vi "Destroy_Tree.vi"(8 "error in (no error)":errorcluster, 10 "Delete Tree Items? (F)":bool, 11 "Tree_LVOOP in":refnum<class "Tree Class.lvclass">) -> (0 "error out":errorcluster)   [LabVIEW 2012, in "Tree Tools.lvlib" / "Tree Class.lvclass"]
uses:
  Tree Class.lvclass
  Tree Class.lvclass/Tree Class.ctl
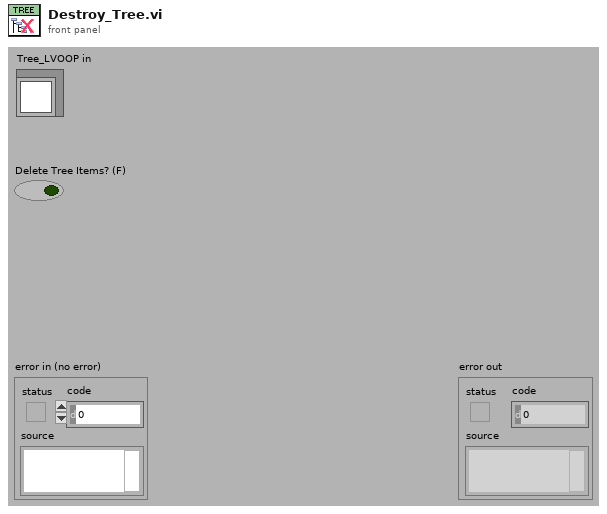
[diagram p1: front panel]
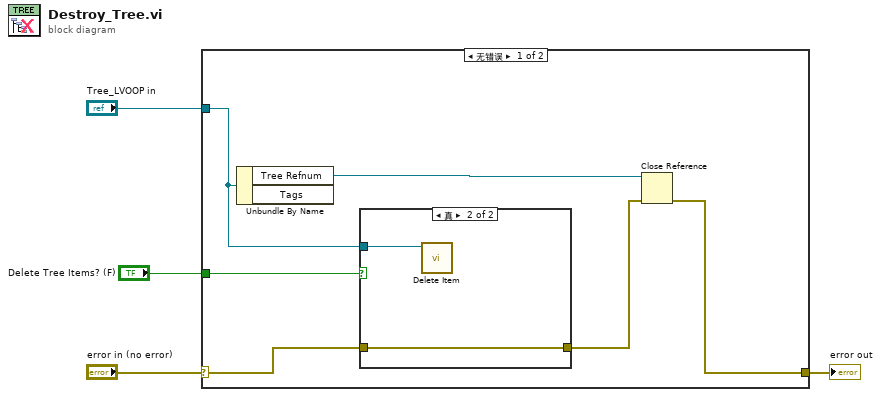
[diagram p0: block diagram]
diagram:
  n1 = case shown="无错误" "error in (no error)" {
    selector: "error in (no error)" -> [w7 w14]
    tunnel: [w9 w14] -> w3
    tunnel: "Tree_LVOOP in" -> [w5 _]
    tunnel: "Delete Tree Items? (F)" -> [w8 _]
    frame No Error {
      n2 = Unbundle By Name(w5) -> ("Tree Refnum"=w10:refnum<vi>)  [unwired: 1 out]
      n3 = case shown="真" w8 {
        tunnel: w7 -> [w11 w13]
        tunnel: [w11 w13] -> w6
        tunnel: w5 -> [_ w12]
        frame False {
        }
        frame True {
          n4 = call-dynamic "Delete Item.vi"("Tree_LVOOP in"=w12) -> ()  [unwired: 4 in, 7 out]
        }
      }
      n5 = Close Reference(reference=w10, error in (no error)=w6) -> (error out=w9:errorcluster)
    }
    frame Error {
    }
  }
  "error out" <- w3
